vi "Fetch Data From DB.vi"(8 "error in (no error)":errorcluster, 9 "Multicolumn Listbox 2":refnum<vi>, 10 "End Time":timestamp, 11 "Start Time":timestamp) -> (0 "error out 2":errorcluster, 2 "Result Set":string[][](table) caption="Result Set (from first statement with results)", 3 "Column Names":string[](array[string]))   [LabVIEW 2020, in "DataBase.lvlib"]
uses:
  DataBase.lvlib
  <vilib>/drjdpowell/SQLite Library/SQL Connection/Open (path).vi
  <vilib>/drjdpowell/SQLite Library/SQL Connection/Open (string).vi
  <vilib>/AdvancedString/Path To Command Line String.vi
  <vilib>/drjdpowell/SQLite Library/SQL Connection/Execute SQL.vi
  <vilib>/drjdpowell/SQLite Library/SQL Connection/Connection.lvclass
  <vilib>/drjdpowell/SQLite Library/SQLite.lvlib
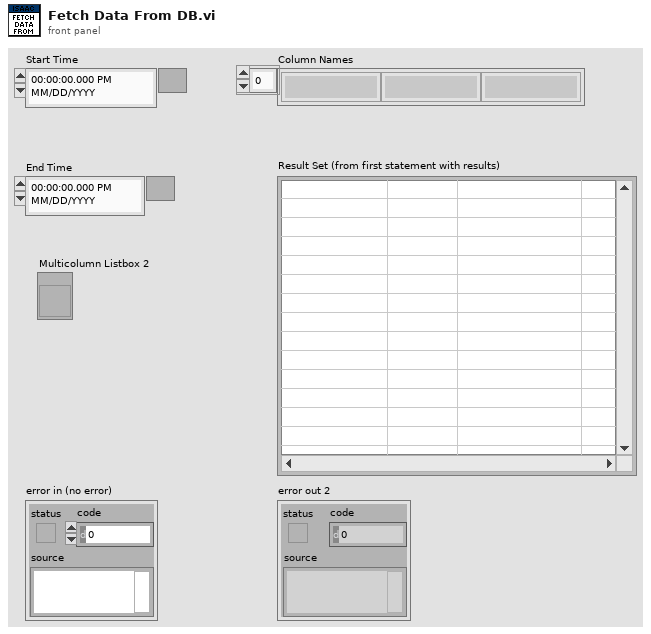
[diagram p1: front panel]
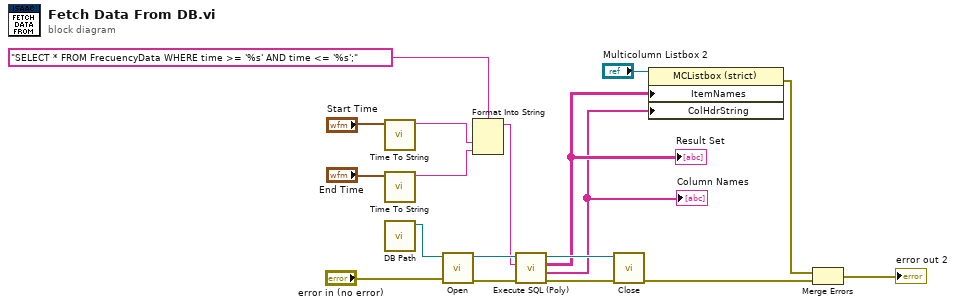
[diagram p0: block diagram]
diagram:
  n1 = call "Time To String.vi"("Time"="Start Time") -> ("date/time string"=w13:string)  [unwired: 10 in]
  n2 = call "Time To String.vi"("Time"="End Time") -> ("date/time string"=w12:string)  [unwired: 10 in]
  n3 = call "DB Path.vi"() -> ("appended path"=w8:path)  [unwired: 11 in]
  n4 = call-poly <vilib>:"Open.vi"("error in (no error)"="error in (no error)", "db file"=w8) -> ("error out"=w18:errorcluster, "SQLite Connection"=w15:refnum<class "Connection.lvclass">)  [unwired: 8 in]
  n5 = Format Into String(format string="SELECT * FROM FrecuencyData WHERE time >= '%s' AND time <= '%s';", w13, w12) -> (resulting string=w1:string)  [unwired: 2 in, 1 out]
  n6 = call-poly <vilib>:"Execute SQL (Poly).vi"("error in (no error)"=w18, "SQL"=w1, "SQLite Connection in"=w15) -> ("error out"=w16:errorcluster, "Column Names"=w5:string[], "Result Set"=w6:string[][], "SQLite Connection"=w17:refnum<class "Connection.lvclass">)  [unwired: 5 in]
  "Result Set" <- w6
  "Column Names" <- w5
  n7 = call-dynamic "Close.vi"("error in (no error)"=w16, "SQLite Connection in"=w17) -> ("error out"=w4:errorcluster)  [unwired: 9 in]
  n8 = property class="MCListbox (strict)"(reference="Multicolumn Listbox 2", "ItemNames"=w6, "ColHdrString"=w5) -> (error out=w3:errorcluster)  [unwired: 1 in, 1 out]
  n9 = Merge Errors(w3, w4) -> (→"error out 2":errorcluster)
